vi "myFreqGroup.vi"(4 "是否需要dq排频":bool, 8 "基波频率":u32=50, 9 "最大同时扫频数":u32=7, 11 "freqs":i32[](array[numeric])) -> (0 "freqs ind group":i32[][](array[numeric]), 1 "freqs index":i32[][](array[numeric]), 2 "freqs group":i32[][](array[numeric]))   [LabVIEW 2024]
doc: "若允许多频点注入，根据 1D freqs 生成解耦的频率组 2D freqs_group，每行为一组频率。\n如果不允许，生成时每行只放s一个频点。\n\n伴生的 freqs_index 与 freqs_ind_group 分别是从 freqs 到 freqs_group，以及反向\n寻址时的对应索引 2D 数组。\n\n当需要正负序（前级输入频率中有部分负频率）的时候，输出中的正负频率是混在一起的。\n也许你会担心，但放心吧，正负序不怕这个。"
uses:
  a1369902-94b3-47df-bc2f-fc5e996f6c32.vi
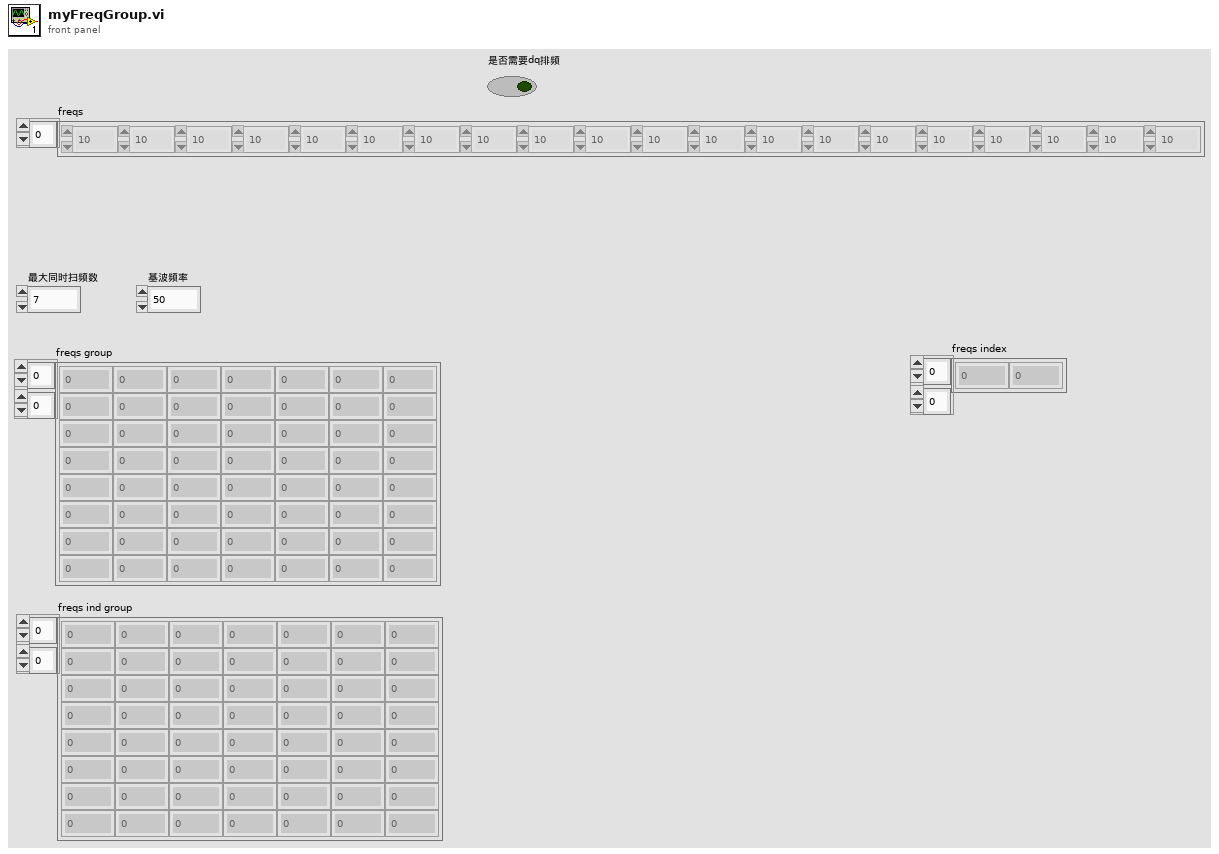
[diagram p1: front panel]
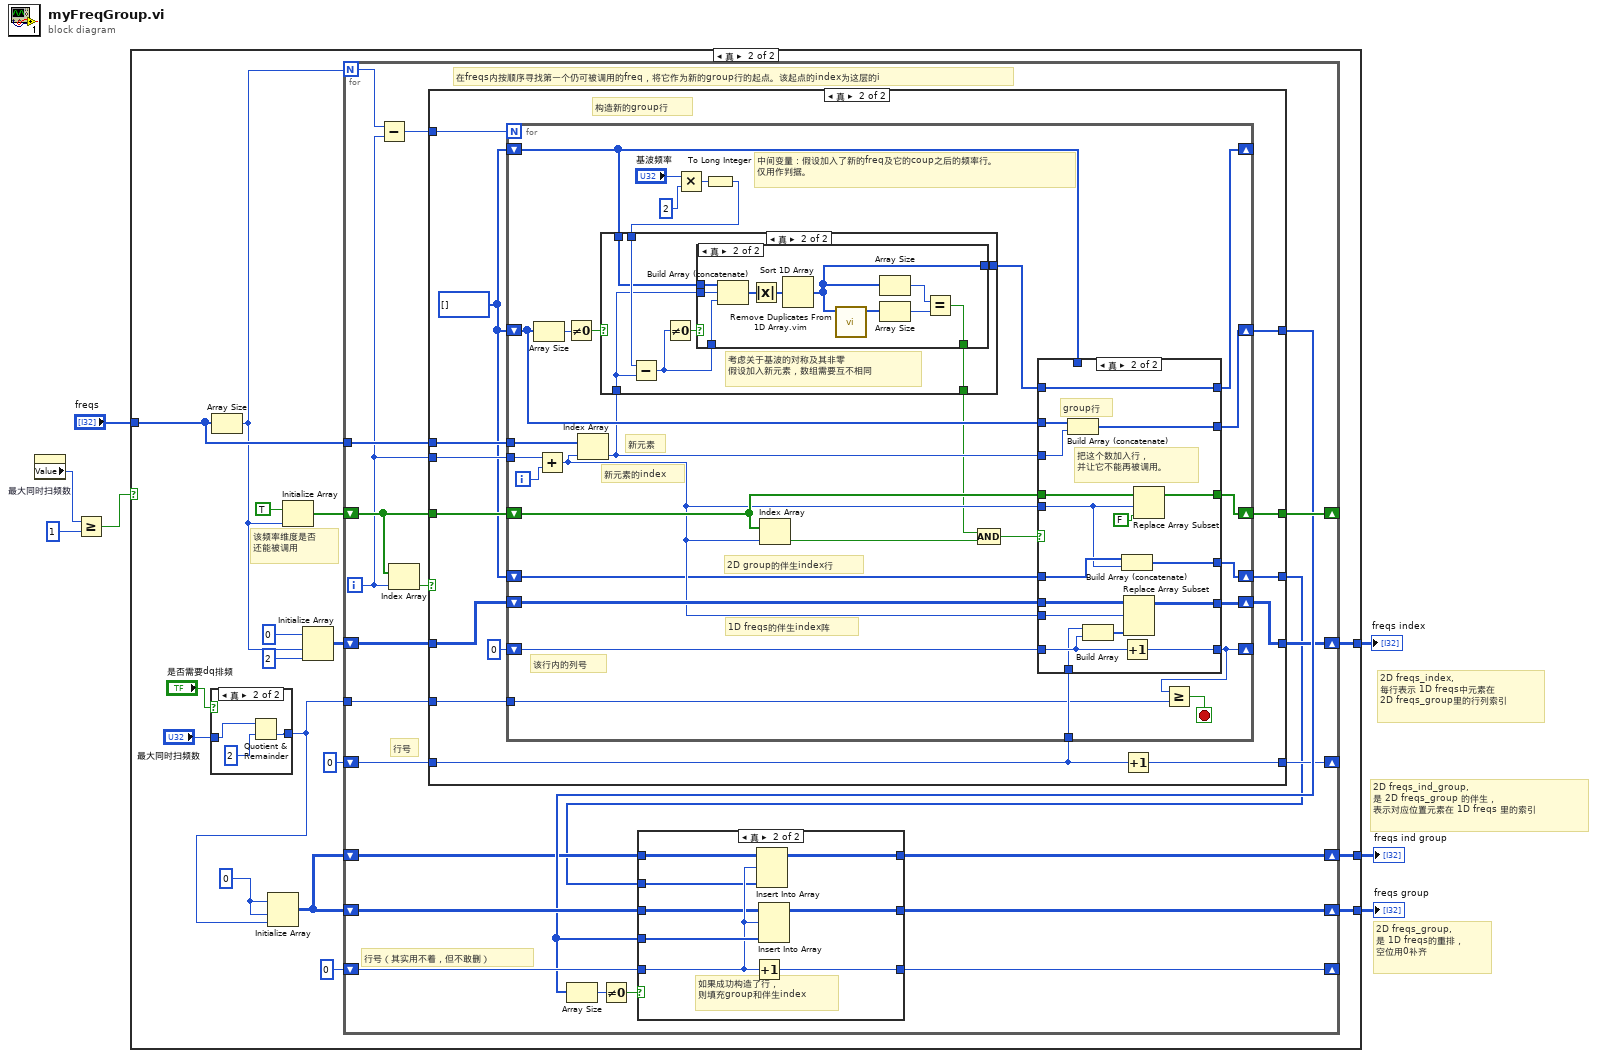
[diagram p0: block diagram]
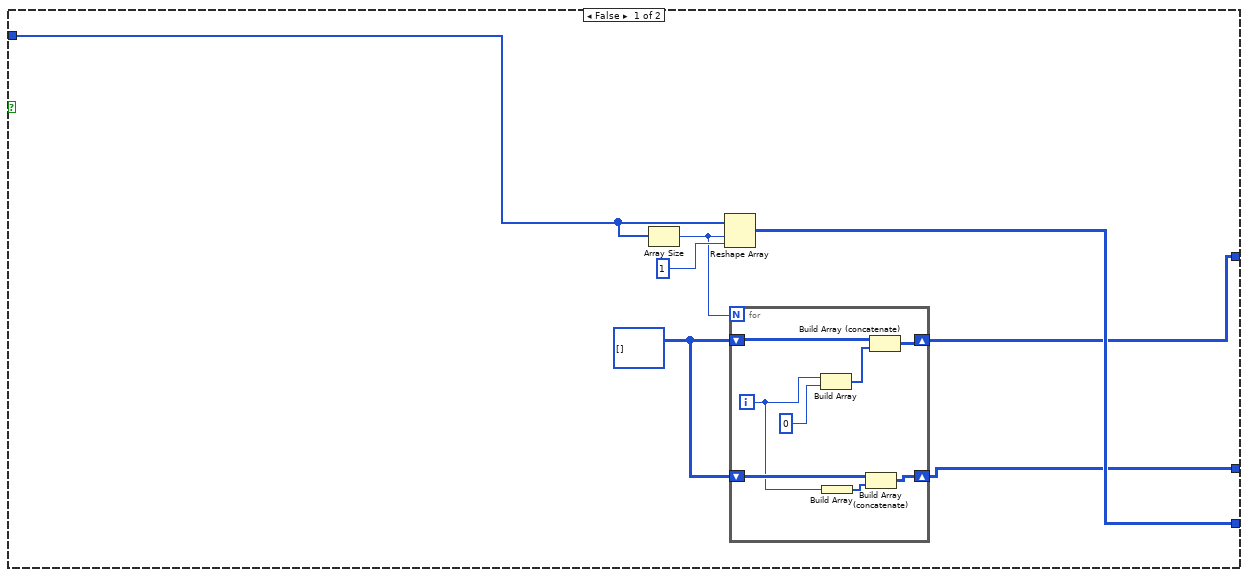
[diagram p2: hidden frame]
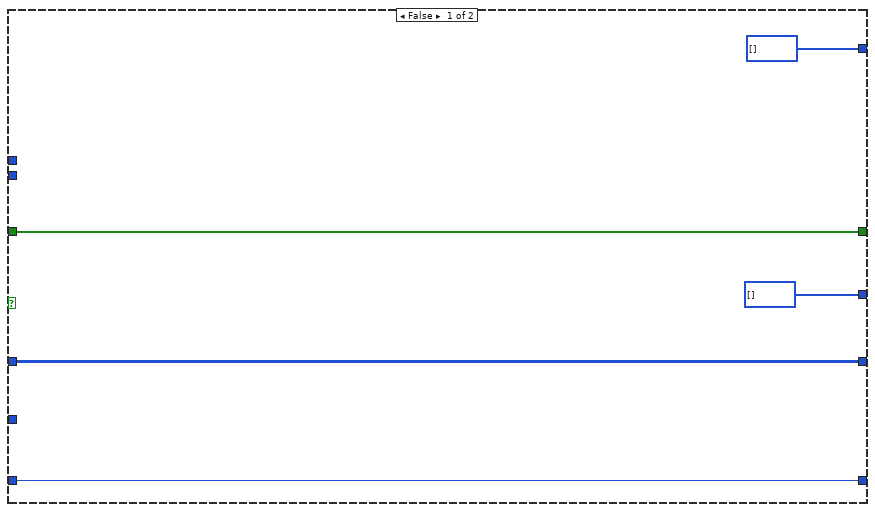
[diagram p5: hidden frame]
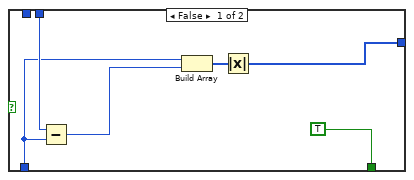
[diagram p6: hidden frame]
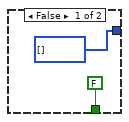
[diagram p7: hidden frame]
diagram:
  # "2D freqs_ind_group,\n是 2D freqs_group 的伴生，\n表示对应位置元素在 1D freqs 里的索引"
  # "2D freqs_group,\n是 1D freqs的重排，\n空位用0补齐"
  # "2D freqs_index,\n每行表示 1D freqs中元素在\n2D freqs_group里的行列索引"
  n1 = property on="最大同时扫频数" class="DigNum (严格)"() -> ("Value"=w3:u32)  [unwired: 2 in, 2 out]
  n2 = Greater Or Equal?(x=w3, y=1) -> (x >= y?=w1:bool)
  n3 = case shown="真" w1 {
    tunnel: [w13 w36] -> w7
    tunnel: "freqs" -> [w12 w35]
    tunnel: [w10 w34] -> w6
    tunnel: [w8 w28] -> w5
    frame False {
      w9 = i32[][] []
      n4 = Array Size(array=w12) -> (size(s)=w11:i32)
      n5 = Reshape Array(w12, w11, 1) -> (w13:i32[][])
      n6 = for {
        N: w11 -> [_]
        shift-right: [w20] -> w10
        shift-left: w9 -> [w21]
        shift-right: [w17] -> w8
        shift-left: w9 -> [w18]
        i -> [w16]
        n7 = Build Array(w16, 0) -> (w22:i32[])
        n8 = Build Array(w16) -> (w15:i32[])
        n9 = Build Array (concatenate)(w18, w15) -> (w17:i32[][])
        n10 = Build Array (concatenate)(w21, w22) -> (w20:i32[][])
      }
    }
    frame True {
      w26 = 0
      # "该频率维度是否\n还能被调用"
      n11 = case shown="真" "是否需要dq排频" {
        tunnel: "最大同时扫频数" -> [w40 w42]
        tunnel: [w40 w41] -> w23
        frame False {
        }
        frame True {
          n12 = Quotient & Remainder(x=w42, y=2) -> (floor(x/y)=w41:u32)  [unwired: 1 out]
        }
      }
      n13 = Array Size(array=w35) -> (size(s)=w33:i32)
      n14 = Initialize Array(w26, w26, w23) -> (w27:i32[][])
      n15 = Initialize Array(TRUE, w33) -> (w38:bool[])
      n16 = Initialize Array(0, w33, 2) -> (w31:i32[][])
      n17 = for {
        N: w33 -> [w55]
        tunnel: w35 -> [w65]
        shift-right: [w57] -> w36
        shift-left: w27 -> [w60]
        shift-right: [w63] -> _
        shift-left: w38 -> [w53]
        shift-right: [w58] -> _
        shift-left: 0 -> [w59]
        shift-right: [w51] -> w34
        shift-left: w31 -> [w52]
        shift-right: [w48] -> _
        shift-left: 0 -> [w49]
        shift-right: [w47] -> w28
        shift-left: w27 -> [w46]
        tunnel: w23 -> [w44]
        i -> [w50]
        # "行号（其实用不着，但不敢删）"
        # "行号"
        # "在freqs内按顺序寻找第一个仍可被调用的freq，将它作为新的group行的起点。该起点的index为这层的i"
        n18 = Subtract(x=w55, y=w50) -> (x-y=w64:i32)
        n19 = Index Array(array=w53, index=w50) -> (element=w54:bool)
        n20 = case shown="真" w54 {
          tunnel: w65 -> [_ w95]
          tunnel: w53 -> [w81 w93]
          tunnel: w64 -> [_ w83]
          tunnel: w50 -> [_ w94]
          tunnel: [w81 w92] -> w63
          tunnel: [i32[] [] w91] -> w56
          tunnel: w52 -> [w79 w90]
          tunnel: [w79 w89] -> w51
          tunnel: w49 -> [w78 w87]
          tunnel: [w78 w86] -> w48
          tunnel: [i32[] [] w84] -> w45
          tunnel: w44 -> [_ w82]
          frame False {
          }
          frame True {
            w85 = i32[] []
            # "构造新的group行"
            n21 = for {
              N: w83 -> [_]
              tunnel: w95 -> [w125]
              shift-right: [w116] -> w91
              shift-left: w85 -> [w119]
              tunnel: w94 -> [w124]
              shift-right: [w122] -> w92
              shift-left: w93 -> [w115]
              shift-right: [w117] -> _
              shift-left: w85 -> [w118]
              shift-right: [w112] -> w89
              shift-left: w90 -> [w113]
              shift-right: [w100] -> _
              shift-left: 0 -> [w101]
              tunnel: w87 -> [w110]
              shift-right: [w108] -> w84
              shift-left: w85 -> [w109]
              tunnel: w82 -> [w96]
              i -> [w123]
              stop <- w99 stop-if-true
              # "该行内的列号"
              # "1D freqs的伴生index阵"
              # "2D group的伴生index行"
              # "中间变量：假设加入了新的freq及它的coup之后的频率行。\n仅用作判据。"
              # "新元素"
              # "新元素的index"
              n22 = Array Size(array=w119) -> (size(s)=w121:i32)
              n23 = Add(x=w124, y=w123) -> (x+y=w111:i32)
              n24 = Not Equal To 0?(x=w121) -> (x != 0?=w120:bool)
              n25 = Index Array(array=w125, index=w111) -> (element=w114:i32)
              n26 = Multiply(x="基波频率", y=2) -> (x*y=w107:u32)
              n27 = To Long Integer(number=w107) -> (32bit integer=w104:i32)
              n28 = case shown="真" w120 {
                tunnel: [TRUE w133] -> w103
                tunnel: w118 -> [_ w137]
                tunnel: w104 -> [w130 w138]
                tunnel: w114 -> [w127 w136]
                tunnel: [w128 w132] -> w97
                frame False {
                  n29 = Subtract(x=w130, y=w127) -> (x-y=w126:i32)
                  n30 = Build Array(w127, w126) -> (w129:i32[])
                  n31 = Absolute Value(x=w129) -> (abs(x)=w128:i32[])
                }
                frame True {
                  # "考虑关于基波的对称及其非零\n假设加入新元素，数组需要互不相同"
                  n32 = Subtract(x=w138, y=w136) -> (x-y=w135:i32)
                  n33 = Not Equal To 0?(x=w135) -> (x != 0?=w134:bool)
                  n34 = case shown="真" w134 {
                    tunnel: w137 -> [_ w150]
                    tunnel: w136 -> [_ w149]
                    tunnel: w135 -> [_ w147]
                    tunnel: [FALSE ("布尔") w141] -> w133
                    tunnel: [i32[] [] w144] -> w132
                    frame False {
                    }
                    frame True {
                      n35 = Build Array (concatenate)(w150, w149, w147) -> (w148:i32[])
                      n36 = Absolute Value(x=w148) -> (abs(x)=w146:i32[])
                      n37 = Sort 1D Array(array=w146) -> (sorted array=w144:i32[])
                      n38 = call "Remove Duplicates From 1D Array.vim"("array"=w144) -> ("array with duplicates removed"=w145:i32[])  [unwired: 10 in]
                      n39 = Array Size(array=w144) -> (size(s)=w143:i32)
                      n40 = Array Size(array=w145) -> (size(s)=w142:i32)
                      n41 = Equal?(x=w143, y=w142) -> (x = y?=w141:bool)
                    }
                  }
                }
              }
              n42 = Index Array(array=w115, index=w111) -> (element=w98:bool)
              n43 = Compound Arithmetic op=AND ("复合运算")(w103, w98) -> (w102:bool)
              n44 = case shown="真" w102 {
                tunnel: w119 -> [w156 w169]
                tunnel: w114 -> [_ w168]
                tunnel: [w156 w170] -> w116
                tunnel: w115 -> [w155 w173]
                tunnel: w111 -> [_ w158]
                tunnel: [w155 w171] -> w122
                tunnel: w118 -> [w154 _]
                tunnel: [w154 w157] -> w117
                tunnel: w113 -> [w152 w167]
                tunnel: [w152 w166] -> w112
                tunnel: w111 -> [_ w165]
                tunnel: w101 -> [w153 w162]
                tunnel: [w153 w163] -> w100
                tunnel: w110 -> [_ w161]
                tunnel: w109 -> [w151 w160]
                tunnel: [w151 w159] -> w108
                tunnel: w97 -> [_ w157]
                frame False {
                }
                frame True {
                  # "group行"
                  # "把这个数加入行，\n并让它不能再被调用。"
                  n45 = Build Array (concatenate)(w169, w168) -> (w170:i32[])
                  n46 = Build Array(w161, w162) -> (w164:i32[])
                  n47 = Build Array (concatenate)(w160, w158) -> (w159:i32[])
                  n48 = Increment(x=w162) -> (x+1=w163:i32)
                  n49 = Replace Array Subset(array=w167, new element=w164, index (row)=w165) -> (w166:i32[][])  [unwired: 1 in]
                  n50 = Replace Array Subset(array=w173, new element=FALSE, index=w158) -> (w171:bool[])
                }
              }
              n51 = Greater Or Equal?(x=w100, y=w96) -> (x >= y?=w99:bool)
            }
            n52 = Increment(x=w87) -> (x+1=w86:i32)
          }
        }
        n53 = Array Size(array=w56) -> (size(s)=w62:i32)
        n54 = Not Equal To 0?(x=w62) -> (x != 0?=w61:bool)
        n55 = case shown="真" w61 {
          tunnel: w60 -> [w67 w70]
          tunnel: w56 -> [_ w74]
          tunnel: w59 -> [w68 w72]
          tunnel: [w68 w76] -> w58
          tunnel: [w67 w75] -> w57
          tunnel: [w66 w73] -> w47
          tunnel: w46 -> [w66 w69]
          tunnel: w45 -> [_ w71]
          frame False {
          }
          frame True {
            # "如果成功构造了行，\n则填充group和伴生index"
            n56 = Increment(x=w72) -> (x+1=w76:i32)
            n57 = Insert Into Array(array=w69, index (row)=w72, new element=w71) -> (w73:i32[][])  [unwired: 1 in]
            n58 = Insert Into Array(array=w70, index (row)=w72, new element=w74) -> (w75:i32[][])  [unwired: 1 in]
          }
        }
      }
    }
  }
  "freqs group" <- w7
  "freqs index" <- w6
  "freqs ind group" <- w5
